vi "ReadPWMConfig(SubVI).vi"(8 "error in (no error)":errorcluster, 11 "appended path":path) -> (0 "error out":errorcluster, 3 "PWM Setting":T1={"DIO_EF_CLOCK1_DIVISOR"=16, "DIO_EF_CLOCK1_ROLL_VALUE"=25000, "DIO#_EF_INDEX"=0, "DIO#_EF_OPTIONS"=1, "DIO#_EF_CONFIG_A"=6250})   [LabVIEW 2020]
uses:
  LJ PWM Setting.ctl
  <vilib>/Utility/file.llb/Read Delimited Spreadsheet (string).vi
  <vilib>/addons/_JKI.lib/Serialization/JSON/JKI JSON Serialization.lvlib
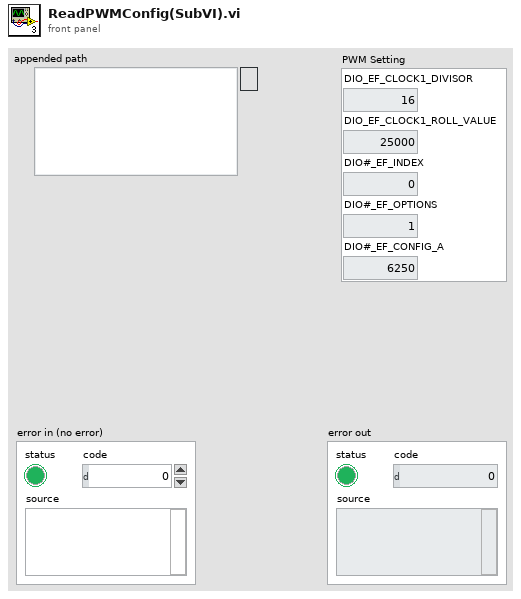
[diagram p1: front panel]
types:
  T1 = typedef "LJ PWM Setting.ctl" = cluster{"DIO_EF_CLOCK1_DIVISOR":i16, "DIO_EF_CLOCK1_ROLL_VALUE":i32, "DIO#_EF_INDEX":i16, "DIO#_EF_OPTIONS":i16, "DIO#_EF_CONFIG_A":i32}
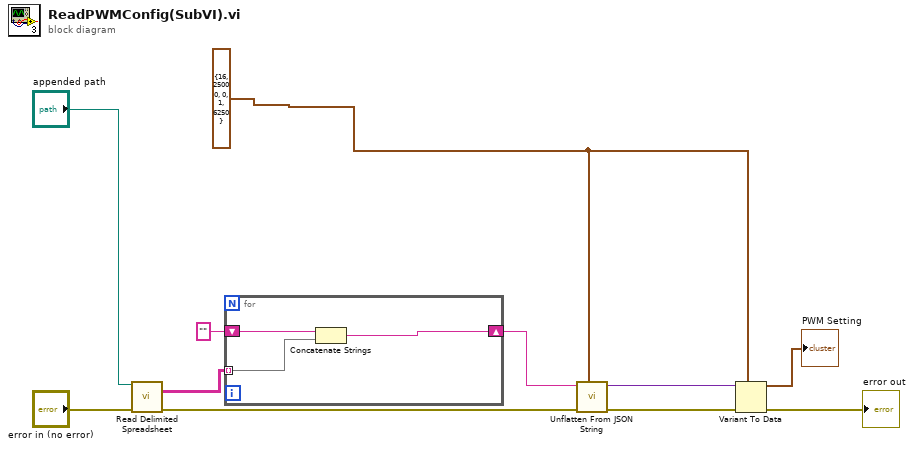
[diagram p0: block diagram]
diagram:
  w1 = T1 {"DIO_EF_CLOCK1_DIVISOR"=16, "DIO_EF_CLOCK1_ROLL_VALUE"=25000, "DIO#_EF_INDEX"=0, "DIO#_EF_OPTIONS"=1, "DIO#_EF_CONFIG_A"=6250} ("PWM setting")
  n1 = call-poly <vilib>:"Read Delimited Spreadsheet.vi"("file path (dialog if empty)"="appended path", "error in (no error)"="error in (no error)") -> ("all rows"=w4:string[][], "error out"=w9:errorcluster)  [unwired: 8 in, 4 out]
  n2 = for {
    tunnel: w4 -> [w14] mode=indexing
    shift-right: [w12] -> w7
    shift-left: "" -> [w13]
    n3 = Concatenate Strings(w13, w14) -> (w12:string)
  }
  n4 = call <vilib>:"Unflatten From JSON String.vi"("Type and Defaults"=w1, "error in"=w9, "JSON String"=w7) -> ("error out"=w10:errorcluster, "Variant"=w6:variant)  [unwired: 7 in]
  n5 = Variant To Data(error in=w10, type=w1, Variant=w6) -> (data=→"PWM Setting":T1, error out=→"error out":errorcluster)
